vi "Read User Timestamps FIFO.vi"(8 "error in (no error)":errorcluster, 11 "FPGA Ref in":refnum<k20>) -> (0 "error out":errorcluster, 2 "Data":u64[](array[numeric]), 3 "FPGA Ref out":refnum<k20>, 5 "Elements Remaining":u32)   [LabVIEW 2025, in "I2C Bus Monitor.lvclass"]
uses:
  I2C Bus Monitor.lvclass
  <vilib>/Utility/error.llb/Error Cluster From Error Code.vi
  <vilib>/rvi/errors/niLvFpgaAdjustHostInterfaceError.vi
  <vilib>/rvi/interface/nirviMethod/nirviMethod.xnode
  I2C Bus Monitor.lvclass/I2C Bus Monitor.ctl
  <vilib>/FPGAPlugInAG/Dynamic/niLvFpga_ReadFifo_Dynamic.vi
  <vilib>/rvi/errors/niLvFpgaMergeErrorWithErrorCode.vi
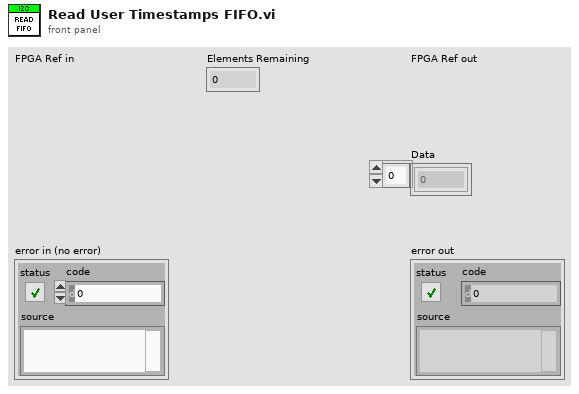
[diagram p1: front panel]
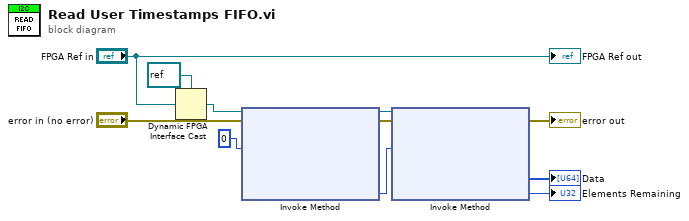
[diagram p0: block diagram]
diagram:
  n1 = Dynamic FPGA Interface Cast(Session In=refnum<k20> refnum ("FPGA VI Reference Out"), Type="FPGA Ref in") -> (Session Out=w8:refnum<k20>)
  n2 = xnode "Invoke Method"("FPGA VI Reference In"=w8, "error in"="error in (no error)", "Number of Elements"=u32 0) -> ("FPGA VI Reference Out"=w2:refnum<k20>, "error out"=w3:errorcluster, "Elements Remaining"=w5:u32)  [unwired: 1 in, 1 out]
  n3 = xnode "Invoke Method"("FPGA VI Reference In"=w2, "error in"=w3, "Number of Elements"=w5) -> ("error out"=→"error out":errorcluster, "Data"=→"Data":u64[], "Elements Remaining"=→"Elements Remaining":u32)  [unwired: 1 in, 1 out]
  "FPGA Ref out" <- "FPGA Ref in"
